vi "index to type.vi"(11 "I32":i32) -> (3 "type":T1)   [LabVIEW 2013, in "data bus tag description.lvclass"]
doc: "A helper function which converts between a standard indexing terminal (I32) and the type enum provided by the framework (U16)."
uses:
  data bus tag description.lvclass
  Data Type.ctl
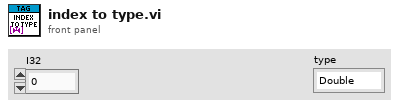
[diagram p1: front panel]
types:
  T1 = typedef "data bus tag description.lvclass/Data Type.ctl" = enum16{"Double", "I64", "Boolean", "Array of Double", "Array of I64", "Variant"}
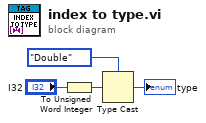
[diagram p0: block diagram]
diagram:
  n1 = To Unsigned Word Integer(number="I32") -> (unsigned 16bit integer=w4:u16)
  n2 = Type Cast(type=Data_Type."Double" ("Data Type"), x=w4) -> (*(type *) &x=→"type":T1)
